vi "Digital Toggle Single.vi"(8 "error in (no error)":errorcluster, 10 "Channel Index":i32, 11 "Digital Writer in":refnum<class "Digital Writer.lvclass">) -> (0 "error out":errorcluster, 3 "Digital Writer out":refnum<class "Digital Writer.lvclass">)   [LabVIEW 2024, in "DAQmx Actor.lvlib" / "Digital Writer.lvclass"]
uses:
  Digital Writer.lvclass
  Digital Writer.lvclass/Digital Writer.ctl
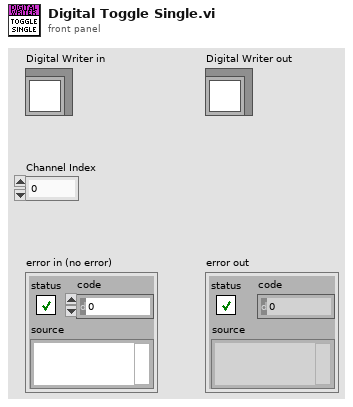
[diagram p1: front panel]
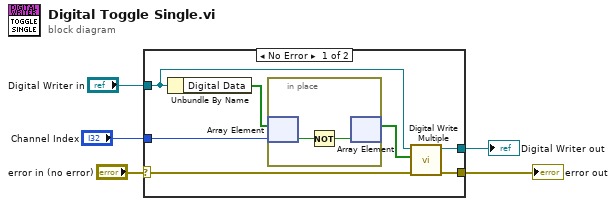
[diagram p0: block diagram]
diagram:
  n1 = case shown="No Error" "error in (no error)" {
    selector: "error in (no error)" -> [w6 w16]
    tunnel: [w7 w16] -> w4
    tunnel: [w8 w15] -> w2
    tunnel: "Digital Writer in" -> [w9 w15]
    tunnel: "Channel Index" -> [w12 _]
    frame No Error {
      n2 = Unbundle By Name(w9) -> ("Digital Data"=w11:bool[])
      n3 = in-place {
        n4 = in-place-array #1(w11, w12) -> (w14:bool)
        n5 = Not(x=w14) -> (.not. x?=w13:bool)
        n6 = in-place-array #1(w13) -> (w10:bool[])  [unwired: 1 out]
      }
      n7 = call-dynamic "Digital Write Multiple.vi"("error in (no error)"=w6, "Digital Data"=w10, "Digital Writer in"=w9) -> ("error out"=w7:errorcluster, "Digital Writer out"=w8:refnum<class "Digital Writer.lvclass">)  [unwired: 7 in]
    }
    frame Error {
    }
  }
  "error out" <- w4
  "Digital Writer out" <- w2
